vi "Read now place.vi"(8 "error in (no error)":errorcluster, 11 "mainclass in":refnum<class "mainclass.lvclass">) -> (0 "error out":errorcluster, 2 "now place":cluster{"x":dbl, "y":dbl}, 3 "mainclass out":refnum<class "mainclass.lvclass">)   [LabVIEW 2013, in "mainclass.lvclass"]
uses:
  mainclass.lvclass
  mainclass.lvclass/mainclass.ctl
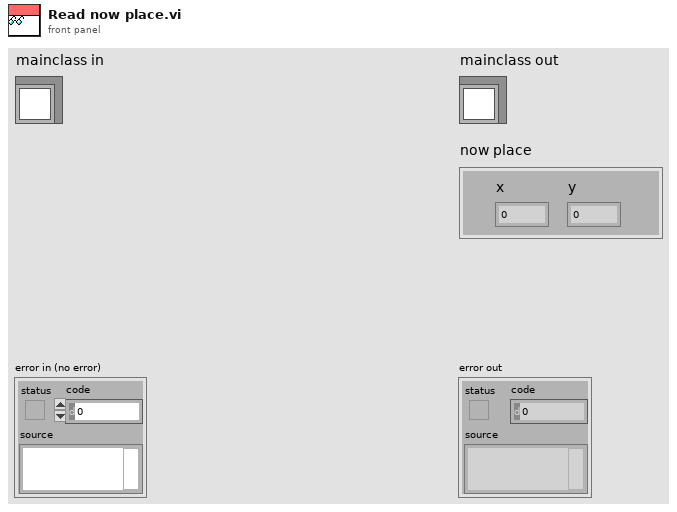
[diagram p1: front panel]
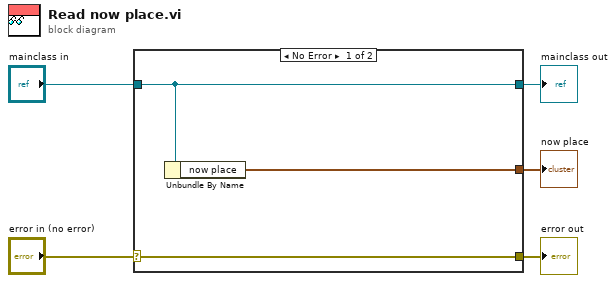
[diagram p0: block diagram]
diagram:
  n1 = case shown="No Error" "error in (no error)" {
    selector: "error in (no error)" -> [w8 w9]
    tunnel: [w8 w9] -> w4
    tunnel: [w7 w10] -> w2
    tunnel: "mainclass in" -> [w7 w10]
    tunnel: [w6 _] -> w1
    frame No Error {
      n2 = Unbundle By Name(w7) -> ("now place"=w6:cluster{"x":dbl, "y":dbl})
    }
    frame Error {
    }
  }
  "error out" <- w4
  "mainclass out" <- w2
  "now place" <- w1
